vi "create polys.vi"(9 "PolyVI Refnum":refnum<vi>, 11 "actual vi":refnum<vi>) -> (3 "error out":errorcluster)   [LabVIEW 2013]
uses:
  source/tag/Data Type.ctl
  generic_type_definition.ctl
  <vilib>/Utility/VariantDataType/Type.ctl
  source/dictionary/look up tag by type.vi
  source/tag/tag descriptor.lvclass
  <vilib>/Utility/VariantDataType/VariantType.lvlib
  source/dictionary/data dictionary.lvclass
panel:
  in  "multiple values":bool
  in  "Data Type":T1
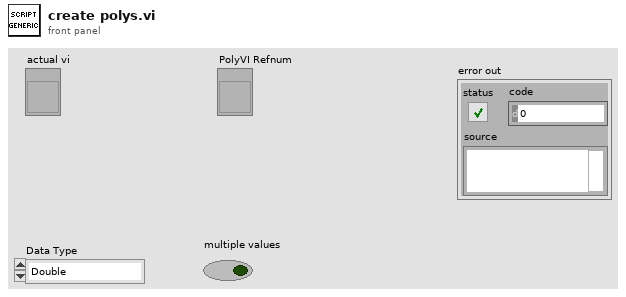
[diagram p1: front panel]
types:
  T1 = typedef "tag bus.lvlib/tag descriptor.lvclass/Data Type.ctl" = enum16{"Double", "Single", "I64", "I32", "I16", "I8", "U64", "U32", "U16", "U8", "Boolean", "String", "Array of Double", "Array of Single", "Array of I64", "Array of I32", "Array of I16", "Array of I8", "Array of U64", "Array of U32", "Array of U16", "Array of U8", "Array of Boolean", "Array of String"}
  T2 = typedef "VariantType.lvlib/Type.ctl" = enum8{"Invalid Type", "Void", "I8", "I16", "I32", "I64", "U8", "U16", "U32", "U64", "Single Float", "Double Float", "Extended Float", "Single Complex", "Double Complex", "Extended Complex", "Enum U8", "Enum U16", "Enum U32", "Enum U64", "Single Float With Unit", "Double Float With Unit", "Extended Float With Unit", "Single Complex with Unit", "Double Complex with Unit", "Extended Complex with Unit", "Boolean", "String", "Path", "Picture", "Tag", "Array", "Cluster", "Variant", "LV Variant", "Waveform", "Timestamp", "Digital Waveform", "Digital Data", "ExpressData", "Refnum", "External Data", "VI", "Poly VI", "LabVIEW Class Instance", "Fixed Point"}
  T3 = typedef "generic_type_definition.ctl" = cluster{"name":string, "Type Enum":T2, "path (cluster)":path, "element type (array)":T2, "cluster of arrays":bool, "array of cluster of arrays":bool}
  T4 = cluster{"VIPath":path, "Menu Name":string, "Selector Name":string}[]
  T5 = cluster{"VIPath":path, "Menu Name":string, "Selector Name":string}
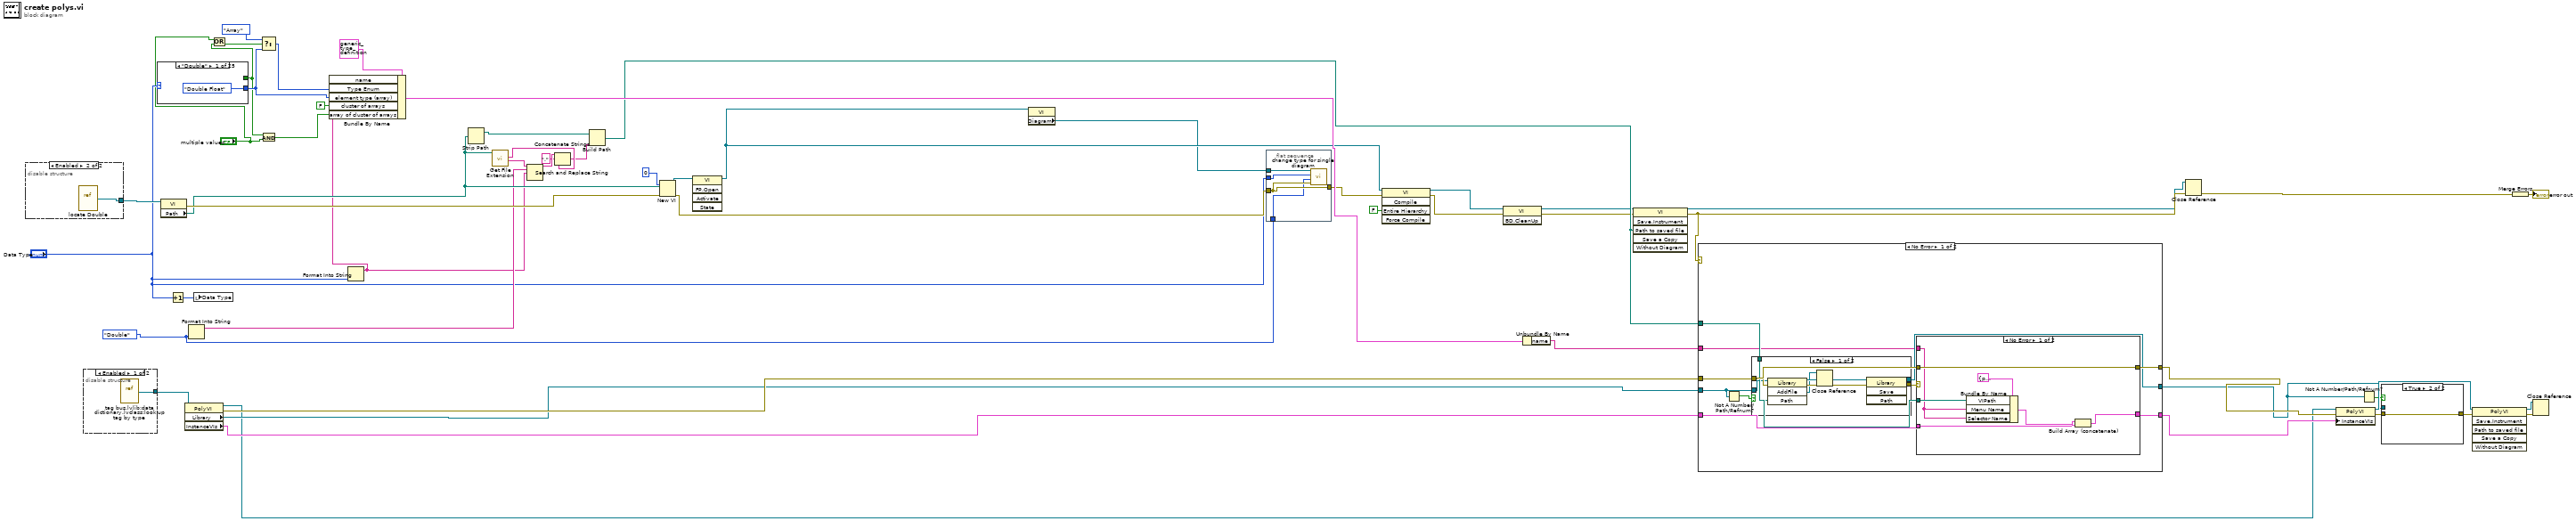
[diagram p0: block diagram]
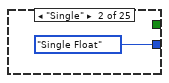
[diagram p2: hidden frame]
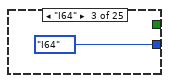
[diagram p3: hidden frame]
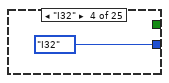
[diagram p4: hidden frame]
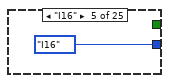
[diagram p5: hidden frame]
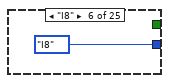
[diagram p6: hidden frame]
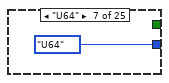
[diagram p7: hidden frame]
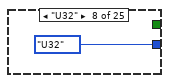
[diagram p8: hidden frame]
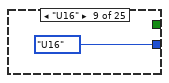
[diagram p9: hidden frame]
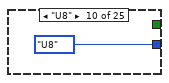
[diagram p10: hidden frame]
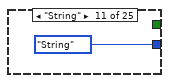
[diagram p11: hidden frame]
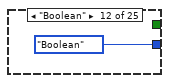
[diagram p12: hidden frame]
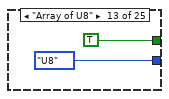
[diagram p13: hidden frame]
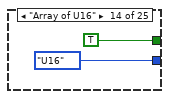
[diagram p14: hidden frame]
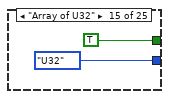
[diagram p15: hidden frame]
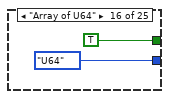
[diagram p16: hidden frame]
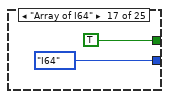
[diagram p17: hidden frame]
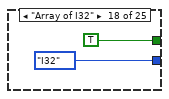
[diagram p18: hidden frame]
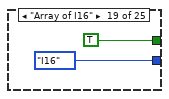
[diagram p19: hidden frame]
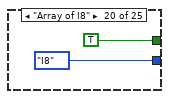
[diagram p20: hidden frame]
diagram:
  w4 = Data_Type."Double" ("element")
  n1 = disable-structure shown="Enabled" {
    disable-tunnel: ["actual vi" w57] -> w37
    frame Disabled {
    }
    frame Enabled {
      n2 = vi-ref "locate Double.vi"() -> (w57:refnum<vi>)
    }
  }
  n3 = disable-structure shown="Enabled" {
    disable-tunnel: [w58 "PolyVI Refnum"] -> w53
    frame Enabled {
      n4 = vi-ref "tag bus.lvlib:data dictionary.lvclass:look up tag by type.vi"() -> (w58:refnum<vi>)
    }
    frame Disabled {
    }
  }
  n5 = case shown="\"Double\"" "Data Type" {
    tunnel: [Type."Double Float" ("Type Enum") Type."Single Float" ("Type Enum") Type."I64" ("Type Enum") Type."I32" ("Type Enum") Type."I16" ("Type Enum") Type."I8" ("Type Enum") Type."U64" ("Type Enum") Type."U32" ("Type Enum") Type."U16" ("Type Enum") Type."U8" ("Type Enum") Type."String" ("Type Enum") Type."Boolean" ("Type Enum") Type."U8" ("Type Enum") Type."U16" ("Type Enum") Type."U32" ("Type Enum") Type."U64" ("Type Enum") Type."I64" ("Type Enum") Type."I32" ("Type Enum") Type."I16" ("Type Enum") Type."I8" ("Type Enum") Type."Double Float" ("Type Enum") Type."Single Float" ("Type Enum") Type."Boolean" ("Type Enum") Type."String" ("Type Enum") Type."Invalid Type" ("Type Enum")] -> w13
    tunnel: [_ _ _ _ _ _ _ _ _ _ _ _ TRUE TRUE TRUE TRUE TRUE TRUE TRUE TRUE TRUE TRUE TRUE TRUE _] -> w8
    frame "Double" {
    }
    frame "Single" {
    }
    frame "I64" {
    }
    frame "I32" {
    }
    frame "I16" {
    }
    frame "I8" {
    }
    frame "U64" {
    }
    frame "U32" {
    }
    frame "U16" {
    }
    frame "U8" {
    }
    frame "String" {
    }
    frame "Boolean" {
    }
    frame "Array of U8" {
    }
    frame "Array of U16" {
    }
    frame "Array of U32" {
    }
    frame "Array of U64" {
    }
    frame "Array of I64" {
    }
    frame "Array of I32" {
    }
    frame "Array of I16" {
    }
    frame "Array of I8" {
    }
    frame "Array of Double" {
    }
    frame "Array of Single" {
    }
    frame "Array of Boolean" {
    }
    frame "Array of String" {
    }
    frame Default {
    }
  }
  n6 = property class="VI"(reference=w37) -> (error out=w55:errorcluster, "Path"=w54:path)  [unwired: 1 in, 1 out]
  n7 = Increment(x="Data Type") -> (x+1=w14:T1)
  n8 = property class="PolyVI"(reference=w53) -> (reference out=w40:refnum<vi>, error out=w51:errorcluster, "Library"=w49:refnum<vi>, "InstanceVIs"=w44:T4)  [unwired: 1 in]
  n9 = Format Into String(w4) -> (resulting string=w36:string)  [unwired: 3 in, 1 out]
  n10 = local write "Data Type"(w14) -> ()
  n11 = Or(x="multiple values", y=w8) -> (x .or. y?=w10:bool)
  n12 = Select(t=Type."Array", s=w10, f=w13) -> (s? t:f=w11:T2)
  n13 = And(x=w8, y="multiple values") -> (x .and. y?=w7:bool)
  n14 = Format Into String("Data Type") -> (resulting string=w33:string)  [unwired: 3 in, 1 out]
  n15 = Bundle By Name(cluster=T3 {"name"="", "Type Enum"=enum."Invalid Type", "path (cluster)"=path "", "element type (array)"=enum."Invalid Type", "cluster of arrays"=FALSE, "array of cluster of arrays"=FALSE}, "name"=w33, "Type Enum"=w11, "element type (array)"=w13, "cluster of arrays"=FALSE, "array of cluster of arrays"=w7) -> (w34:T3)
  n16 = Strip Path(path=w54) -> (stripped path=w18:path)  [unwired: 1 out]
  n17 = call <vilib>:"Get File Extension.vi"("file"=w54) -> ("filename without extension"=w23:string, "lowercase file extension"=w20:string)  [unwired: 7 in, 2 out]
  n18 = Search and Replace String(input string=w23, search string=w36, replace string=w33) -> (result string=w22:string)  [unwired: 5 in, 3 out]
  n19 = Concatenate Strings(w22, "." ("string"), w20) -> (w19:string)
  n20 = Build Path(base path=w18, name or relative path=w19) -> (appended path=w24:path)
  n21 = New VI(7:u32 0 ("options"), 8:w55, 10:w54) -> (0:w30:errorcluster, 3:w31:refnum<vi>)  [unwired: 4 in]
  n22 = invoke class="VI" method="FP.Open"(reference=w31) -> (reference out=w17:refnum<vi>)  [unwired: 4 in, 4 out]
  n23 = property class="VI"(reference=w17) -> ("Diagram"=w15:refnum<vi>)  [unwired: 1 in, 2 out]
  n24 = flat-sequence {
    tunnel: w30 -> [w100]
    tunnel: [w100] -> w16
    tunnel: w15 -> [w99]
    tunnel: "Data Type" -> [w98]
    tunnel: w4 -> [w97]
    frame #0 {
      n25 = call "change type for single diagram.vi"("error in (no error)"=w100, "old type"=w97, "new type"=w98, "Diagram in"=w99) -> ()  [unwired: 8 in]
    }
  }
  n26 = invoke class="VI" method="Compile"(reference=w17, error in=w16, "Entire Hierarchy"=FALSE ("Compile Entire Hierarchy (F)")) -> (reference out=w2:refnum<vi>, error out=w28:errorcluster)  [unwired: 2 in, 3 out]
  n27 = invoke class="VI" method="BD.CleanUp"(reference=w2, error in=w28) -> (reference out=w1:refnum<vi>, error out=w3:errorcluster)  [unwired: 1 in, 1 out]
  n28 = Unbundle By Name(w34) -> ("name"=w25:string)
  n29 = invoke class="VI" method="Save.Instrument"(reference=w1, error in=w3, "Path to saved file"=w24) -> (reference out=w26:refnum<vi>, error out=w27:errorcluster)  [unwired: 3 in, 4 out]
  n30 = case shown="No Error" w27 {
    tunnel: [w109 w133] -> w46
    tunnel: w51 -> [w108 w133]
    tunnel: w49 -> [w102 w132]
    tunnel: [w105 w132] -> w39
    tunnel: [w106 w131] -> w41
    tunnel: w44 -> [w107 w131]
    tunnel: w24 -> [w104 _]
    tunnel: w25 -> [w103 _]
    frame No Error {
      n31 = Not A Number/Path/Refnum?(number/path/refnum=w102) -> (NaN/Path/Refnum?=w101:bool)
      n32 = case shown="False" w101 {
        tunnel: [w115 w121] -> w110
        tunnel: w108 -> [w114 w121]
        tunnel: [w113 w120] -> w105
        tunnel: w104 -> [w112 _]
        tunnel: w102 -> [w111 w120]
        frame False {
          n33 = invoke class="Library" method="AddFile"(reference=w111, error in=w114, "Path"=w112) -> (reference out=w118:refnum<vi>, error out=w119:errorcluster, "AddFile"=w116:refnum<vi>)  [unwired: 1 in, 1 out]
          n34 = Close Reference(reference=w116, error in (no error)=w119) -> (error out=w117:errorcluster)
          n35 = invoke class="Library" method="Save"(reference=w118, error in=w117) -> (reference out=w113:refnum<vi>, error out=w115:errorcluster)  [unwired: 2 in, 2 out]
        }
        frame True {
        }
      }
      n36 = case shown="No Error" w110 {
        tunnel: [w128 w130] -> w109
        tunnel: w108 -> [w128 w130]
        tunnel: w107 -> [w124 w129]
        tunnel: [w126 w129] -> w106
        tunnel: w104 -> [w123 _]
        tunnel: w103 -> [w122 _]
        frame No Error {
          n37 = Bundle By Name(cluster=T5 {"VIPath"=path "", "Menu Name"="", "Selector Name"=""}, "VIPath"=w123, "Menu Name"=w122, "Selector Name"=w122) -> (w125:T5)
          n38 = Build Array (concatenate)(w124, w125) -> (w126:T4)
        }
        frame Error {
        }
      }
    }
    frame Error {
    }
  }
  n39 = Close Reference(reference=w26, error in (no error)=w27) -> (error out=w52:errorcluster)
  n40 = property class="PolyVI"(reference=w40, error in=w46, "InstanceVIs"=w41) -> (reference out=w42:refnum<vi>, error out=w43:errorcluster)
  n41 = Not A Number/Path/Refnum?(number/path/refnum=w39) -> (NaN/Path/Refnum?=w38:bool)
  n42 = case shown="True" w38 {
    tunnel: [w137 w139] -> w45
    tunnel: w43 -> [w135 w139]
    tunnel: w39 -> [w134 _]
    frame False {
      n43 = invoke class="Library" method="Save"(reference=w134, error in=w135) -> (reference out=w136:refnum<vi>, error out=w138:errorcluster)  [unwired: 2 in, 2 out]
      n44 = Close Reference(reference=w136, error in (no error)=w138) -> (error out=w137:errorcluster)
    }
    frame True {
    }
  }
  n45 = invoke class="PolyVI" method="Save.Instrument"(reference=w42, error in=w45) -> (reference out=w47:refnum<vi>, error out=w48:errorcluster)  [unwired: 4 in, 4 out]
  n46 = Merge Errors(w52) -> (→"error out":errorcluster)
  n47 = Close Reference(reference=w47, error in (no error)=w48) -> ()  [unwired: 1 out]
